vi "Key - Read to Spreadsheet String.vi"(8 "error in (no error)":errorcluster, 9 "String in":string, 10 "Control in":refnum<vi>, 11 "ini File Ref num":T1) -> (0 "error out":errorcluster, 1 "String out":string)   [LabVIEW 2013]
uses:
  <vilib>/Utility/config.llb/Config Data RefNum.ctl
  <vilib>/Utility/config.llb/Read Key (String).vi
  <vilib>/Utility/config.llb/NI_LVConfig.lvlib
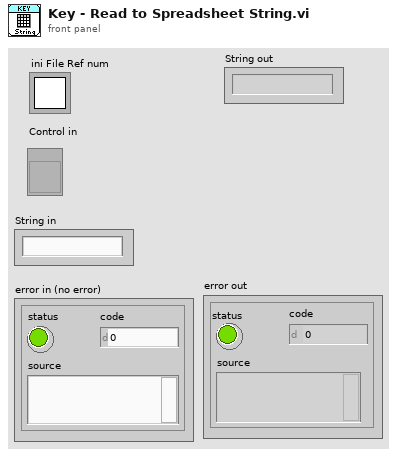
[diagram p1: front panel]
types:
  T1 = typedef "NI_LVConfig.lvlib/Config Data RefNum.ctl" = refnum<k1>
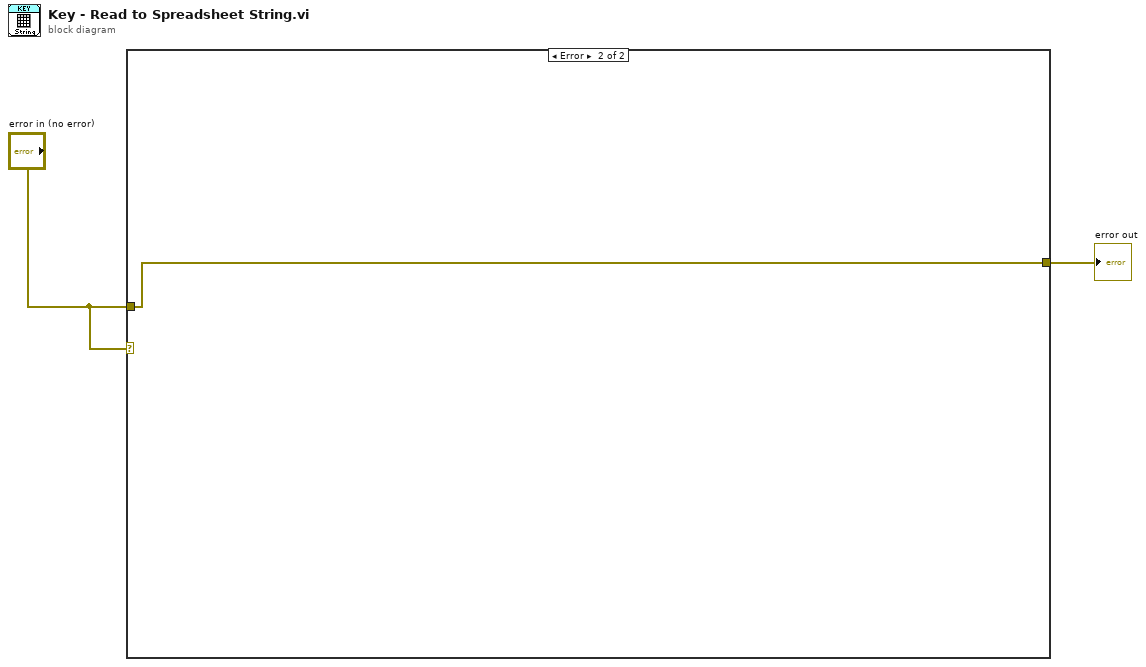
[diagram p0: block diagram]
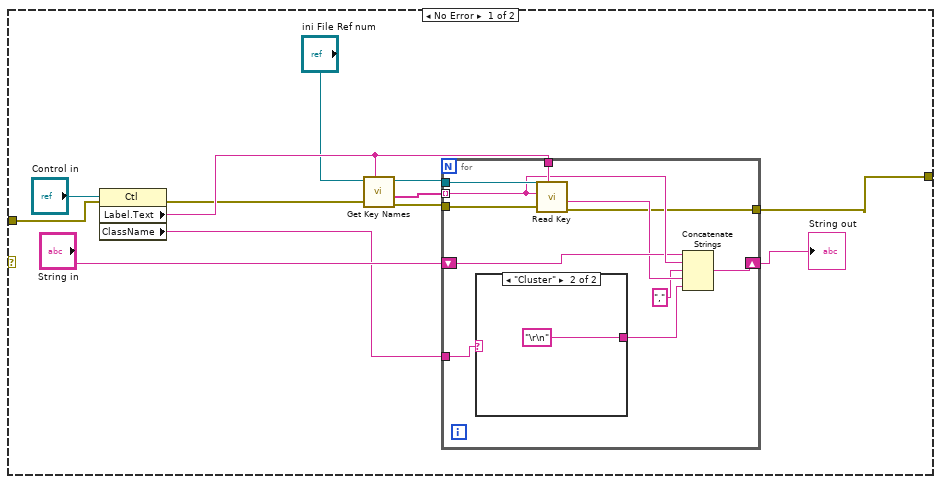
[diagram p2: hidden frame]
diagram:
  n1 = case shown="Error" "error in (no error)" {
    tunnel: [w6 w27] -> w2
    tunnel: "error in (no error)" -> [w4 w27]
    frame No Error {
      n2 = property class="Ctl"(reference="Control in", error in=w4) -> (error out=w3:errorcluster, "Label.Text"=w11:string, "ClassName"=w5:string)  [unwired: 1 out]
      n3 = call <vilib>:"Get Key Names.vi"("section"=w11, "error in (no error)"=w3, "refnum"="ini File Ref num") -> ("error out"=w12:errorcluster, "key names"=w8:string[], "refnum out"=w9:T1)  [unwired: 5 in, 1 out]
      n4 = for {
        tunnel: w9 -> [w25]
        tunnel: w12 -> [w24]
        tunnel: w8 -> [w22] mode=indexing
        tunnel: w11 -> [w23]
        shift-right: [w20] -> w13
        shift-left: "String in" -> [w21]
        tunnel: [w17] -> w6
        tunnel: w5 -> [w16]
        n5 = case shown="\"Cluster\"" w16 {
          tunnel: [_ "\r\n"] -> w15
          frame "False", Default {
          }
          frame "Cluster" {
          }
        }
        n6 = call-poly <vilib>:"Read Key.vi"("section"=w23, "error in (no error)"=w24, "key"=w22, "refnum"=w25) -> ("error out"=w17:errorcluster, "value"=w19:string)  [unwired: 4 in, 2 out]
        n7 = Concatenate Strings(w21, w22, "," ("string"), w19, w15) -> (w20:string)
      }
      "String out" <- w13
    }
    frame Error {
    }
  }
  "error out" <- w2
